vi "Write Multiple to String Log.vi"(10 "Strings to Log":string[](array[string]), 11 "String Control Sink in":refnum<class "String Control Sink.lvclass">) -> (0 "error out":errorcluster, 3 "String Control Sink out":refnum<class "String Control Sink.lvclass">)   [LabVIEW 2019, in "String Control Sink.lvclass"]
uses:
  String Control Sink.lvclass
  String Control Sink.lvclass/String Control Sink.ctl
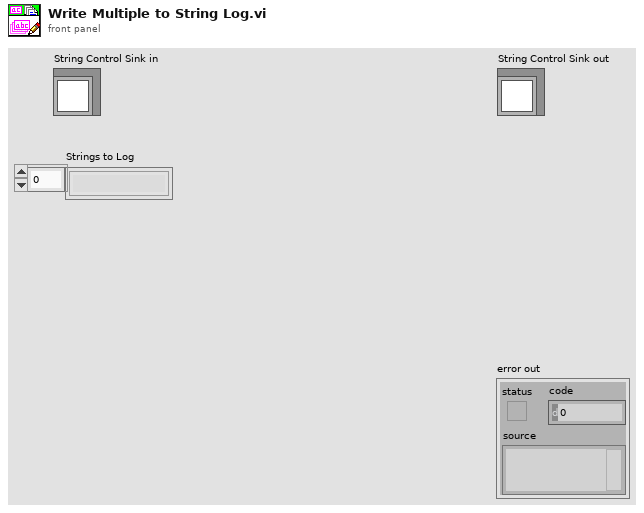
[diagram p1: front panel]
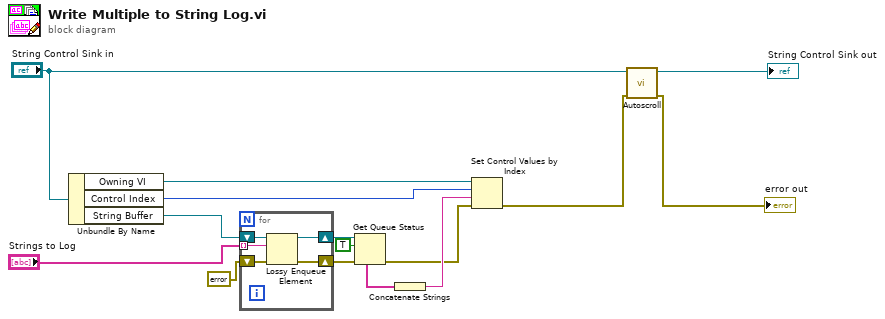
[diagram p0: block diagram]
diagram:
  n1 = Unbundle By Name("String Control Sink in") -> ("Owning VI"=w15:refnum<vi>, "Control Index"=w14:i32, "String Buffer"=w8:refnum<queue>)
  n2 = for {
    tunnel: "Strings to Log" -> [w19] mode=indexing
    shift-right: [w18] -> w5
    shift-left: w8 -> [w20]
    shift-right: [w17] -> w4
    shift-left: errorcluster {"status"=FALSE, "code"=0, "source"=""} ("error out") -> [w16]
    n3 = Lossy Enqueue Element(queue=w20, element=w19, error in (no error)=w16) -> (queue out=w18:refnum<queue>, error out=w17:errorcluster)  [unwired: 2 out]
  }
  n4 = Get Queue Status(queue=w5, return elements? (F)=TRUE, error in (no error)=w4) -> (error out=w1:errorcluster, elements=w2:string[])  [unwired: 6 out]
  n5 = Concatenate Strings(w2) -> (w7:string)
  n6 = Set Control Values by Index(0:w15, 1:w14, 2:w7, 3:w1) -> (11:w10:errorcluster)
  n7 = call "Autoscroll.vi"("error in (no error)"=w10, "String Control Sink in"="String Control Sink in") -> ("error out"=→"error out":errorcluster, "String Control Sink out"=→"String Control Sink out":refnum<class "String Control Sink.lvclass">)  [unwired: 8 in]
